vi "Apply Application Style.vi"(8 "error in (no error)":errorcluster, 10 "VI Refnum":refnum<vi>, 11 "IApplicationStyle in":refnum<class "IApplicationStyle.lvclass">) -> (0 "error out":errorcluster)   [LabVIEW 2017, in "IViewable.lvlib" / "IApplicationStyle.lvclass"]
uses:
  IApplicationStyle.lvclass
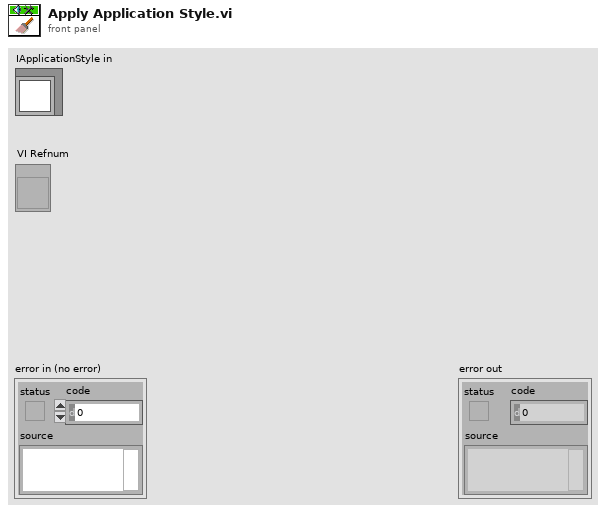
[diagram p1: front panel]
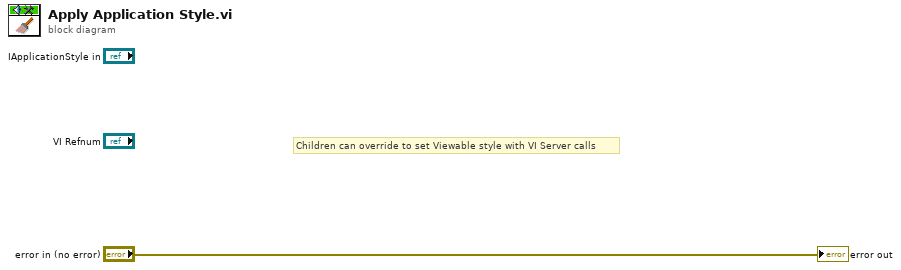
[diagram p0: block diagram]
diagram:
  # "Children can override to set Viewable style with VI Server calls"
  "error out" <- "error in (no error)"
